vi "Test_Sim_SoftFP.vi"(0 "reference in":refnum<class "Test_Sim.lvclass">, 2 "Floating":bool, 5 "error in (no error)":errorcluster) -> (14 "reference out":refnum<class "Test_Sim.lvclass">, 19 "error out":errorcluster)   [LabVIEW 2020, in "Test_Sim.lvlib" / "Test_Sim.lvclass"]
uses:
  Test_Sim.lvclass
  Components/ViPER.lvlibp/ViPER.lvclass
  C:/Projects/Medulla/Presentations/Sydney_LVUG/Demo/Flux_Capacitor_Tester/Components/ViPER.lvlibp/ViPER.lvclass
panel:
  # "Put your FP UI here"
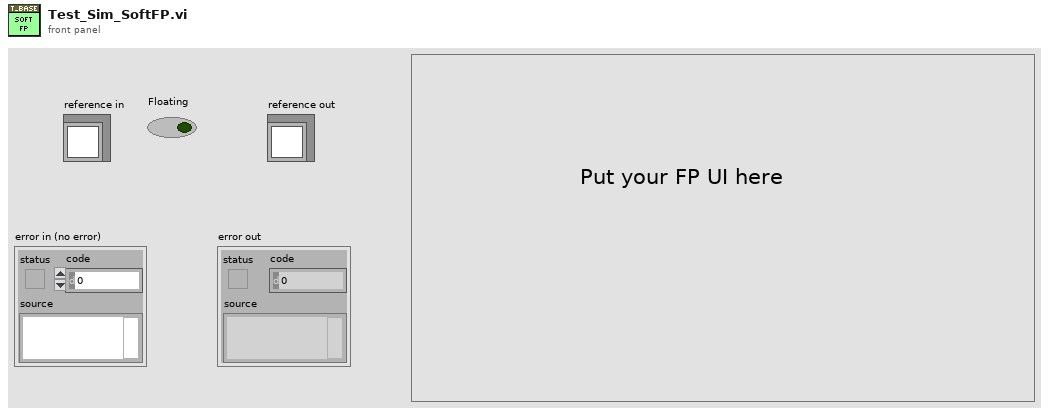
[diagram p1: front panel]
types:
  T1 = enum32{"Invalid", "Standard", "Closed", "Hidden", "Minimized", "Maximized"}
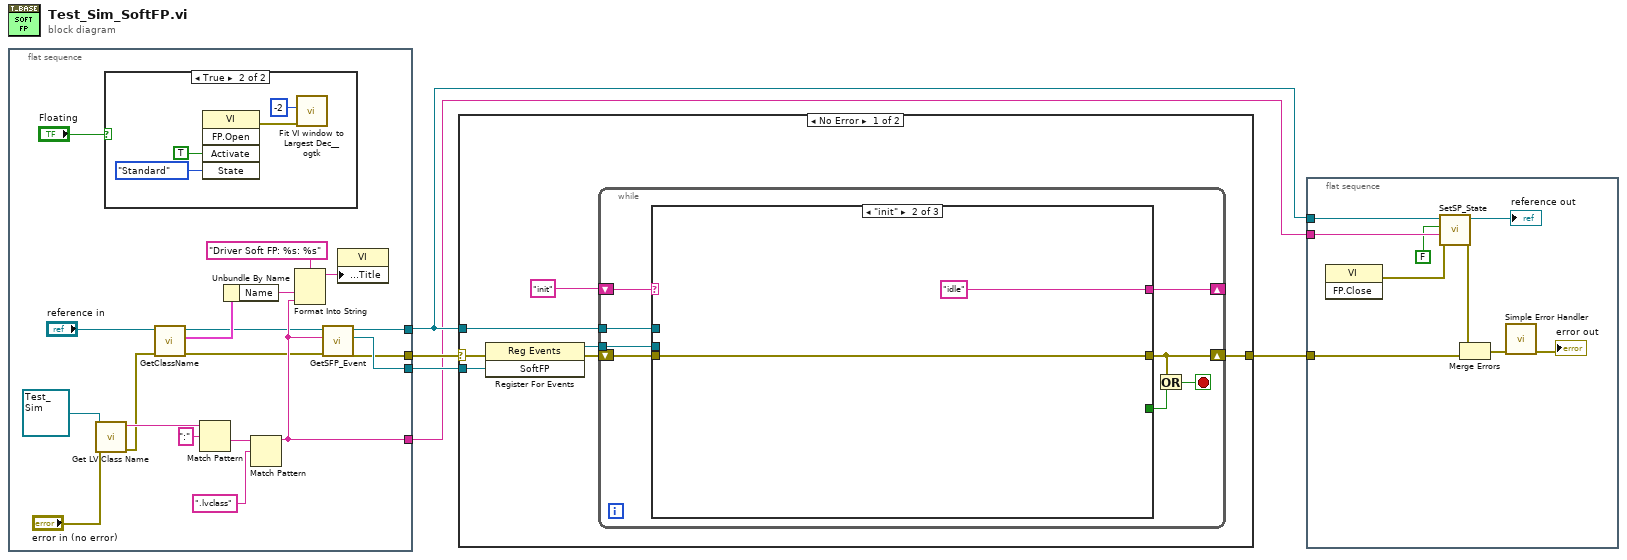
[diagram p0: block diagram]
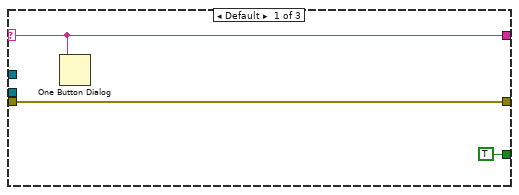
[diagram p3: hidden frame]
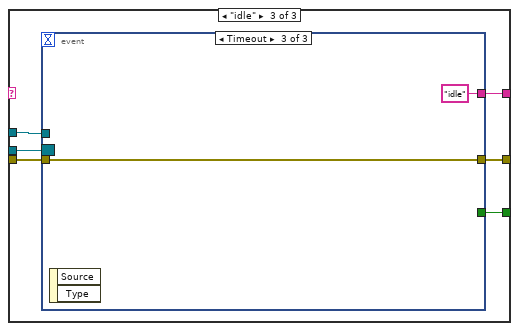
[diagram p4: hidden frame]
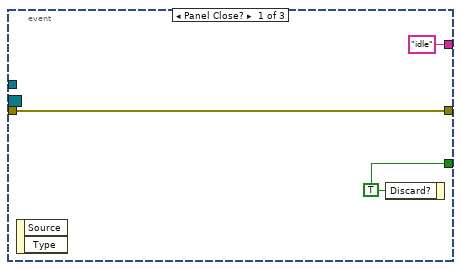
[diagram p5: hidden frame]
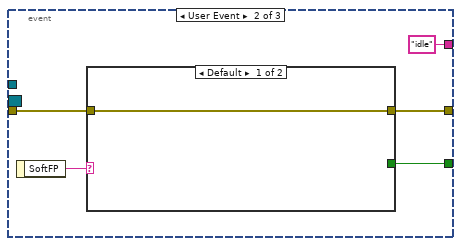
[diagram p6: hidden frame]
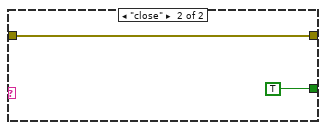
[diagram p7: hidden frame]
diagram:
  n1 = flat-sequence {
    tunnel: [w21] -> w5
    tunnel: [w20] -> w2
    tunnel: [w24] -> w3
    tunnel: [w12] -> w1
    frame #0 {
      n2 = call <vilib>:"Get LV Class Name.vi"("error in (no error)"="error in (no error)", "object"=refnum<class "Test_Sim.lvclass"> refnum ("reference")) -> ("error out"=w11:errorcluster, "class name"=w17:string)  [unwired: 8 in]
      n3 = case shown="True" "Floating" {
        frame False {
        }
        frame True {
          n4 = invoke class="VI" method="FP.Open"("Activate"=TRUE ("Activate?"), "State"=T1."Standard") -> (error out=w25:errorcluster)  [unwired: 3 in, 4 out]
          n5 = call <userlib>:"Fit VI window to Largest Dec__ogtk.vi"("error in (no error)"=w25, "border spacing (2 px)"=-2) -> ()  [unwired: 4 in, 2 out]
        }
      }
      n6 = call "GetClassName.vi"("error in (no error)"=w11, "reference in"="reference in") -> ("error out"=w10:errorcluster, "Details"=w9:cluster{"Name":string, "Class":string}, "reference out"=w7:refnum<class "Test_Sim.lvclass">)  [unwired: 7 in]
      n7 = Match Pattern(string=w17, regular expression=":") -> (after substring=w15:string)  [unwired: 1 in, 3 out]
      n8 = Unbundle By Name(w9) -> ("Name"=w19:string)
      n9 = Match Pattern(string=w15, regular expression=".lvclass") -> (before substring=w12:string)  [unwired: 1 in, 3 out]
      n10 = Format Into String(format string="Driver Soft FP: %s: %s", w19, w12) -> (resulting string=w23:string)  [unwired: 2 in, 1 out]
      n11 = call-dynamic "GetSFP_Event.vi"("error in (no error)"=w10, "Ancestor"=w12, "reference in"=w7) -> ("error out"=w21:errorcluster, "SoftFP"=w24:refnum<user-event>, "reference out"=w20:refnum<class "Test_Sim.lvclass">)  [unwired: 6 in]
      n12 = property class="VI"("Front Panel.Title"=w23) -> ()  [unwired: 2 in, 2 out]
    }
  }
  n13 = case shown="No Error" w5 {
    selector: w5 -> [w33 w68]
    tunnel: [w29 w68] -> w4
    tunnel: w2 -> [w30 _]
    tunnel: w3 -> [w35 _]
    frame No Error {
      n14 = register-events(error in=w33, w35) -> (reference out=w34:refnum<event-registration>, error out=w32:errorcluster)  [unwired: 1 in]
      n15 = while {
        shift-right: [w40] -> w29
        shift-left: w32 -> [w43]
        tunnel: w34 -> [w42]
        tunnel: w30 -> [w41]
        shift-right: [w36] -> _
        shift-left: "init" -> [w37]
        stop <- w39 stop-if-true
        n16 = case shown="\"init\"" w37 {
          selector: w37 -> [w44 _ _]
          tunnel: w43 -> [w45 w47 w54]
          tunnel: w42 -> [_ _ w53]
          tunnel: w41 -> [_ _ w52]
          tunnel: [w45 w47 w51] -> w40
          tunnel: [TRUE ("Discard?") _ w50] -> w38
          tunnel: [w44 "idle" w49] -> w36
          frame Default {
            n17 = One Button Dialog(message=w44) -> ()  [unwired: 1 in, 1 out]
          }
          frame "init" {
          }
          frame "idle" {
            n18 = event shown="[2] Timeout" {
              selector: w53 -> [_ _ _]
              dyn-events: _ -> [_ _ _]
              timeout: _ -> [_ _ _]
              tunnel: w54 -> [w57 w62 w67]
              tunnel: [w57 w60 w67] -> w51
              tunnel: [w56 w59 _] -> w50
              tunnel: w52 -> [_ _ _]
              tunnel: ["idle" "idle" "idle"] -> w49
              event Panel Close? {
                w56 = TRUE ("Discard?")
                n19 = event-data() -> ()  [unwired: 1 in, 2 out]
                n20 = event-data("Discard?"=w56) -> ()  [unwired: 1 in, 1 out]
              }
              event User Event {
                n21 = event-data() -> ("SoftFP"=w61:string)  [unwired: 1 in]
                n22 = case shown="Default" w61 {
                  tunnel: w62 -> [w63 w65]
                  tunnel: [w63 w65] -> w60
                  tunnel: [_ TRUE ("Discard?")] -> w59
                  frame Default {
                  }
                  frame "close" {
                  }
                }
              }
              event Timeout {
                n23 = event-data() -> ()  [unwired: 1 in, 2 out]
              }
            }
          }
        }
        n24 = Or(x=w40, y=w38) -> (x .or. y?=w39:bool)
      }
    }
    frame Error {
    }
  }
  n25 = flat-sequence {
    tunnel: w4 -> [w75]
    tunnel: w2 -> [w70]
    tunnel: w1 -> [w72]
    frame #0 {
      n26 = invoke class="VI" method="FP.Close"() -> (error out=w74:errorcluster)  [unwired: 3 in, 2 out]
      n27 = call "SetSP_State.vi"("error in (no error)"=w74, "Ancestor"=w72, "SP Open"=FALSE, "reference in"=w70) -> ("error out"=w73:errorcluster, "reference out"=→"reference out":refnum<class "Test_Sim.lvclass">)  [unwired: 6 in]
      n28 = Merge Errors(w73, w75) -> (w77:errorcluster)
      n29 = call <vilib>:"Simple Error Handler.vi"("error in (no error)"=w77) -> ("error out"=→"error out":errorcluster)  [unwired: 4 in, 4 out]
    }
  }
